vi "Get Display Data.vi"(8 "error in (no error)":errorcluster, 11 "Base Display Configuration in":refnum<class "Base Display Configuration.lvclass">) -> (0 "error out":errorcluster, 2 "Display Data":T1)   [LabVIEW 2016, in "Assert API Components.lvlib" / "Assert Display.lvlib" / "Main Display.lvlib" / "Base Display Configuration.lvclass"]
uses:
  Base Display Configuration.lvclass
  Components/Display Data.ctl
  Main Display/Display Colours.ctl
  Main Display.lvlib
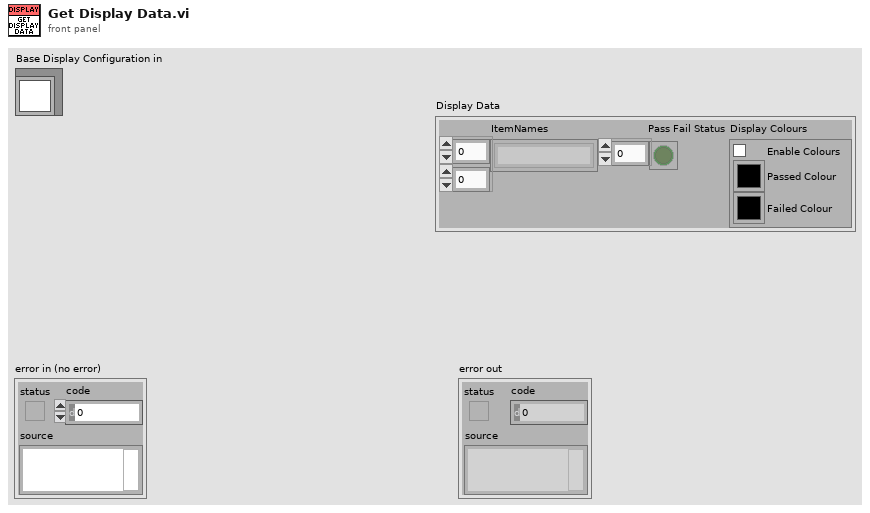
[diagram p1: front panel]
types:
  T1 = typedef "Assert API Components.lvlib/Assert Display.lvlib/Main Display.lvlib/Display Data.ctl" = cluster{"ItemNames":string[][], "Pass Fail Status":bool[], "Display Colours":T2}
  T2 = typedef "Assert API Components.lvlib/Assert Display.lvlib/Main Display.lvlib/Display Colours.ctl" = cluster{"Enable Colours":bool, "Passed Colour":u32, "Failed Colour":u32}
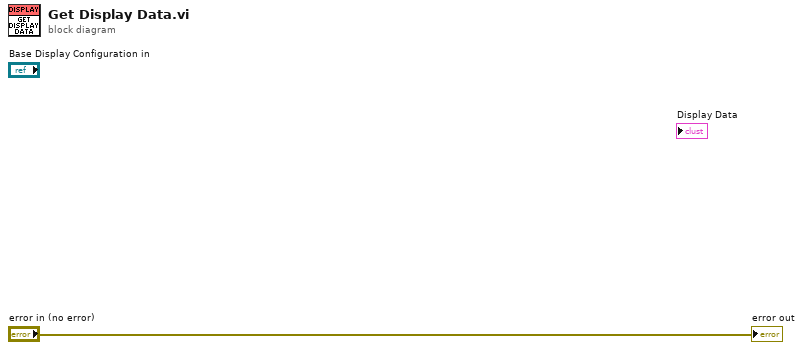
[diagram p0: block diagram]
diagram:
  "error out" <- "error in (no error)"
